vi "Calc - A.vi"(11 "K":dbl) -> (3 "A":dbl)   [LabVIEW 2018, in "Controller (Host).lvlib"]
uses:
  Controller (Host).lvlib
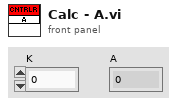
[diagram p1: front panel]
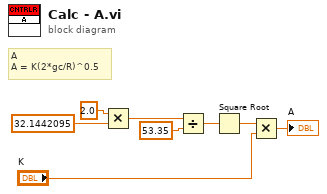
[diagram p0: block diagram]
diagram:
  # "A \nA = K(2*gc/R)^0.5"
  n1 = Multiply(x=2.0, y=32.1442095) -> (x*y=w3:dbl)
  n2 = Divide(x=w3, y=53.35) -> (x/y=w2:dbl)
  n3 = Square Root(x=w2) -> (sqrt(x)=w1:dbl)
  n4 = Multiply(x=w1, y="K") -> (x*y=→"A":dbl)
